vi "Back Propagation.vi"(10 "X Input":dbl[](array[numeric]), 11 "Neuron Stucture In":T1) -> (3 "Neuron Stucture Out":T1)   [LabVIEW 2012]
uses:
  NeuronData.ctl
panel:
  # "Chuck Streb Dec2007"
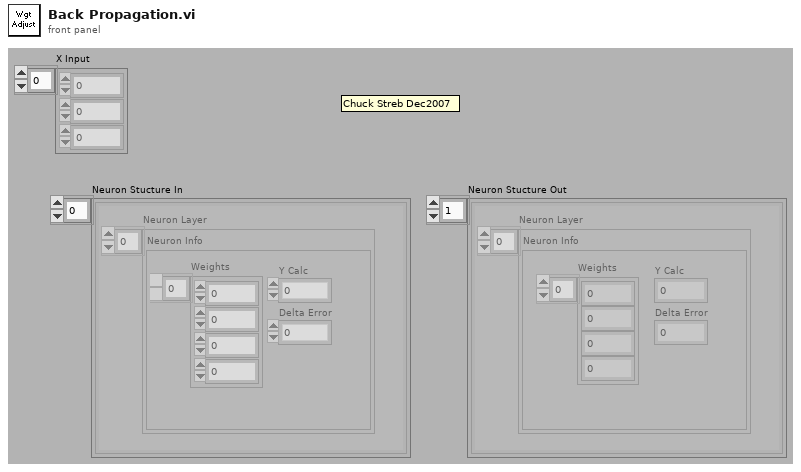
[diagram p1: front panel]
types:
  T1 = typedef "NeuronData.ctl" = cluster{"Neuron Layer":cluster{"Weights":dbl[], "Y Calc":dbl, "Delta Error":dbl}[]}[]
  T2 = cluster{"Weights":dbl[], "Y Calc":dbl, "Delta Error":dbl}[]
  T3 = cluster{"Weights":dbl[], "Y Calc":dbl, "Delta Error":dbl}
  T4 = cluster{"Neuron Layer":cluster{"Weights":dbl[], "Y Calc":dbl, "Delta Error":dbl}[]}
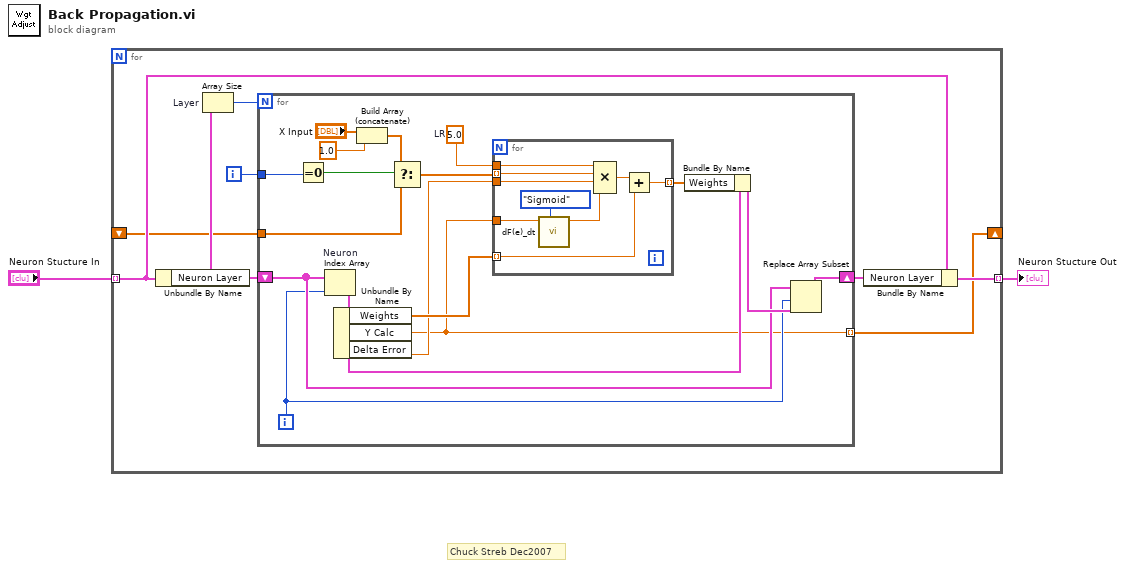
[diagram p0: block diagram]
diagram:
  # "Chuck Streb Dec2007"
  n1 = for {
    tunnel: "Neuron Stucture In" -> [w10] mode=indexing
    tunnel: [w9] -> w1 mode=indexing
    shift-right: [w5] -> _
    shift-left: _ -> [w3]
    i -> [w4]
    n2 = Unbundle By Name(w10) -> ("Neuron Layer"=w8:T2)
    n3 = Array Size "Layer"(array=w8) -> (size(s)=w7:i32)
    n4 = for {
      N: w7 -> [_]
      shift-right: [w20] -> w6
      shift-left: w8 -> [w22]
      tunnel: [w11] -> w5 mode=indexing
      tunnel: w4 -> [w15]
      tunnel: w3 -> [w13]
      i -> [w21]
      w18 = sgl 5.0  # LR
      n5 = Equal To 0?(x=w15) -> (x = 0?=w14:bool)
      n6 = Index Array "Neuron"(array=w22, index=w21) -> (element=w24:T3)
      n7 = Unbundle By Name(w24) -> ("Weights"=w25:dbl[], "Y Calc"=w11:dbl, "Delta Error"=w12:dbl)
      n8 = Build Array (concatenate)("X Input", 1.0) -> (w16:dbl[])
      n9 = Select(t=w16, s=w14, f=w13) -> (s? t:f=w17:dbl[])
      n10 = for {
        tunnel: w18 -> [w36]
        tunnel: w17 -> [w35] mode=indexing
        tunnel: w12 -> [w34]
        tunnel: w11 -> [w32]
        tunnel: w25 -> [w29] mode=indexing
        tunnel: [w28] -> w19 mode=indexing
        n11 = call "dF(e)_dt.vi"("Function"=enum16{"Linear", "Sigmoid", "Tangent hyp."}."Sigmoid", "yout"=w32) -> ("New Weight"=w31:sgl)  [unwired: 9 in]
        n12 = Compound Arithmetic op=MULTIPLY(w36, w35, w34, w31) -> (w30:dbl)
        n13 = Add(x=w30, y=w29) -> (x+y=w28:dbl)
      }
      n14 = Bundle By Name(cluster=w24, "Weights"=w19) -> (w23:T3)
      n15 = Replace Array Subset(array=w22, new element=w23, index=w21) -> (w20:T2)
    }
    n16 = Bundle By Name(cluster=w10, "Neuron Layer"=w6) -> (w9:T4)
  }
  "Neuron Stucture Out" <- w1
